vi "Set Cursor Busy.vi"(8 "error in (no error)":errorcluster, 11 "Panel Actor in":refnum<class "Panel Actor.lvclass">) -> (0 "error out":errorcluster, 2 "Cursor":refnum<class "Cursor.lvclass">)   [LabVIEW 2017, in "MGI-Panel Actor.lvlib" / "Panel Actor.lvclass"]
doc: "Defers updates for the panel.\n\n----\nCopyright: MGI 2018\nAuthor: Derek Trepanier"
uses:
  Panel Actor.lvclass
  panel-manager/Source/Panel Helper/Panel Helper.lvclass
  panel-manager/Source/Cursor/Cursor.lvclass
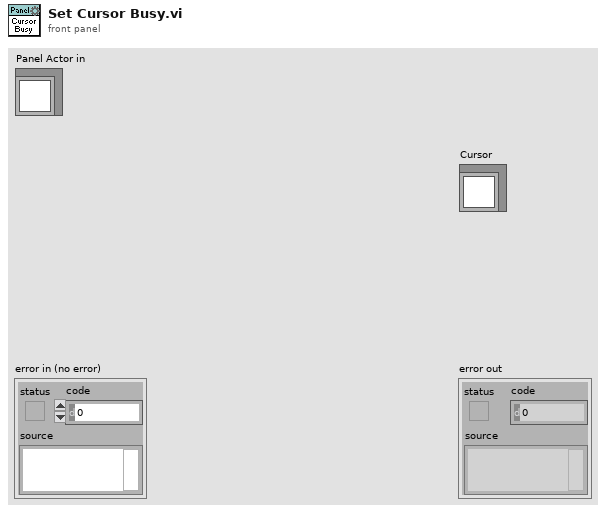
[diagram p1: front panel]
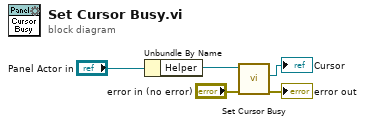
[diagram p0: block diagram]
diagram:
  n1 = Unbundle By Name("Panel Actor in") -> ("Helper"=w4:refnum<class "Panel Helper.lvclass">)
  n2 = call "Set Cursor Busy.vi"("error in (no error)"="error in (no error)", "Panel Helper in"=w4) -> ("error out"=→"error out":errorcluster, "Cursor"=→"Cursor":refnum<class "Cursor.lvclass">)  [unwired: 8 in]
